vi "Wechart Send Message.vi"(8 "error in":errorcluster, 9 "content":string, 10 "Open ID":string, 11 "Token":string="48_KK4v9FCrZjtN20v_jsQ04h-Ab_enIxamJTh8-RmZmdqq_F-XjFkw0ahrX0Lo4peePKKrjuZSgdOCIDaCLMAwgQuxA757qrdiGxoyDd6q0PcdiPV7xYil-UIZ-YgzjJ_sdqpyG85ATqAQj653YMEjAAALZR") -> (0 "error out":errorcluster, 3 "Reply":string)   [LabVIEW 2020]
uses:
  <vilib>/httpClient/POSTBuffer.vi
  <vilib>/httpClient/LabVIEWHTTPClient.lvlib
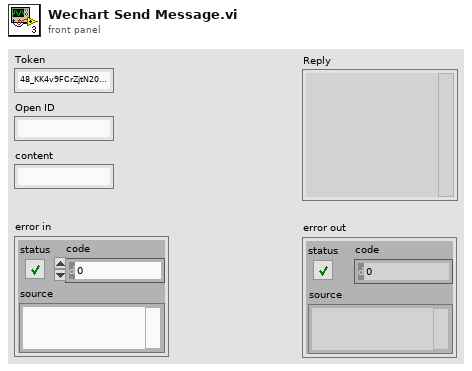
[diagram p1: front panel]
types:
  T1 = cluster{"touser":string, "msgtype":string, "text":cluster{"content":string}}
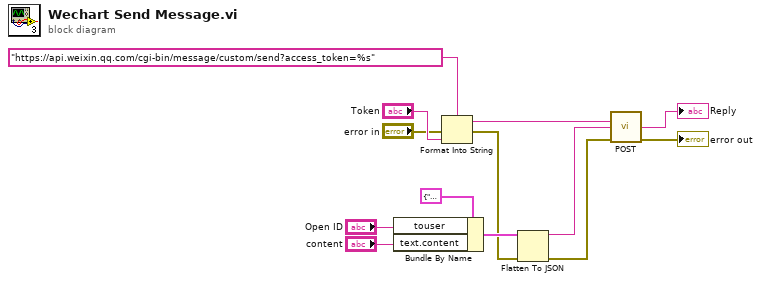
[diagram p0: block diagram]
diagram:
  n1 = Bundle By Name(cluster=T1 {"touser"="o5NgY64UYqTYJlJ02s3ujBymuMNo", "msgtype"="text", "text"={"content"="DEMO"}}, "touser"="Open ID", "text.content"="content") -> (w5:T1)
  n2 = Format Into String(format string="https://api.weixin.qq.com/cgi-bin/message/custom/send?access_token=%s", error in="error in", "Token") -> (resulting string=w12:string, error out=w4:errorcluster)  [unwired: 1 in]
  n3 = Flatten To JSON(anything=w5, error in (no error)=w4) -> (JSON string=w10:string, 11:w3:errorcluster)  [unwired: 1 in]
  n4 = call-poly <vilib>:"POST.vi"("url"=w12, "buffer"=w10, "error in (no error)"=w3) -> ("body"=→"Reply":string, "error out"=→"error out":errorcluster)  [unwired: 9 in, 2 out]
